vi "Set-Get-Wavelength_PM.vi"(0 "instrument handle":refnum<visa-resource-name>, 5 "Wavelength":dbl caption="Wavelength (0.0)", 7 "Sensor Name":string, 9 "Average Count":i32=1 min=1 step=1, 11 "error in (no error)":errorcluster {"code" format="%.0x"}) -> (4 "instrument handle out":refnum<visa-resource-name>, 6 "Wavelength":dbl, 8 "Sensor Name 2":string caption="Sensor Name", 10 "Average Count 2":i32=1 min=1 step=1, 15 "error out":errorcluster)   [LabVIEW 2018]
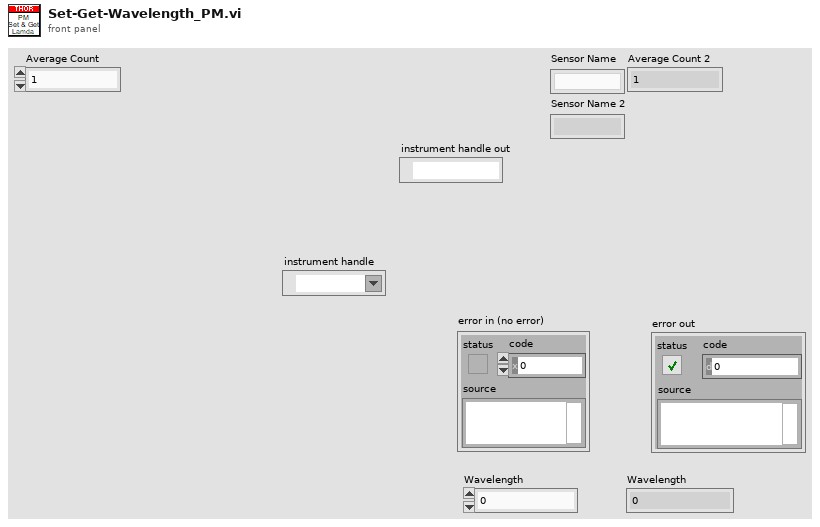
[diagram p1: front panel]
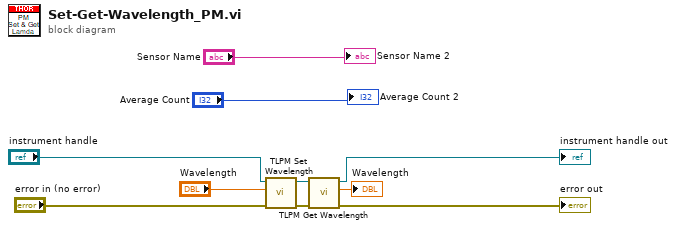
[diagram p0: block diagram]
diagram:
  n1 = call "TLPM Set Wavelength.vi"("error in (no error)"="error in (no error)", "Wavelength (0.0)"="Wavelength", "instrument handle"="instrument handle") -> ("error out"=w3:errorcluster, "instrument handle out"=w6:refnum<visa-resource-name>)  [unwired: 7 in]
  n2 = call "TLPM Get Wavelength.vi"("error in (no error)"=w3, "instrument handle"=w6) -> ("error out"=→"error out":errorcluster, "Wavelength"=→"Wavelength":dbl, "instrument handle out"=→"instrument handle out":refnum<visa-resource-name>)  [unwired: 7 in]
  "Sensor Name 2" <- "Sensor Name"
  "Average Count 2" <- "Average Count"
